vi "LV_client_23.vi"() -> ()   [LabVIEW 2022 SP3]
doc: "Demo VI, client making TCP connection with server on the local port 8089"
panel:
  out "Path to Python script":path
  out "error out":errorcluster
  in  "Stop":bool
  out "Answer":string
  in  "Ping":bool
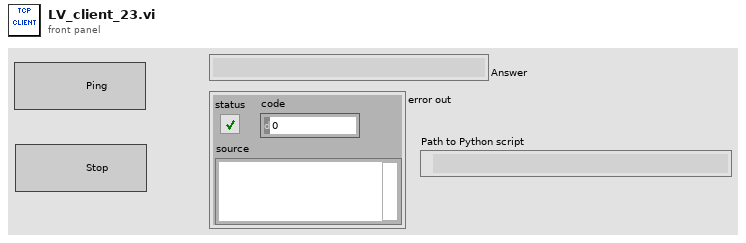
[diagram p1: front panel]
types:
  T1 = enum8{"Enabled", "Disabled", "Disabled and Grayed Out"}
  T2 = enum16{"Standard", "Buffered", "CRLF", "Immediate"}
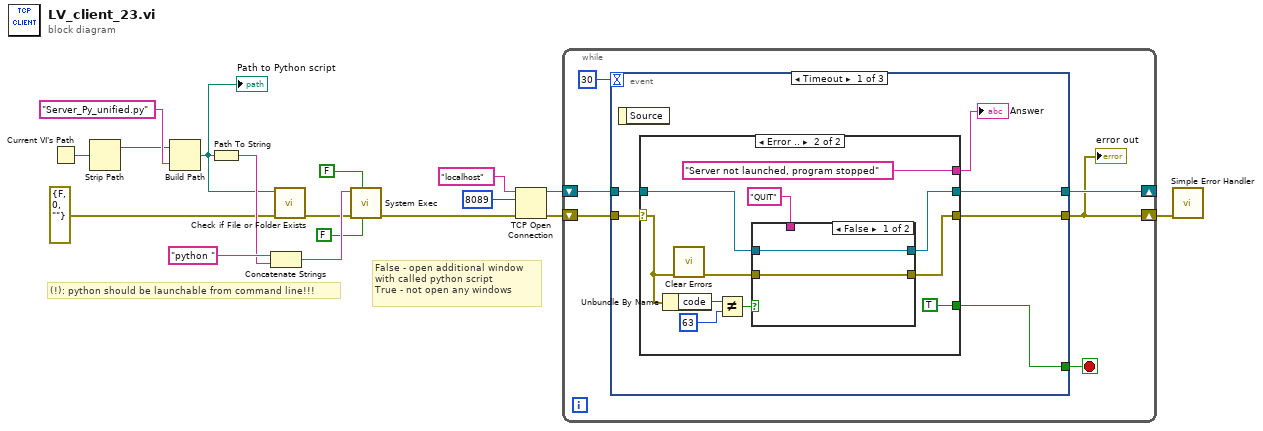
[diagram p0: block diagram]
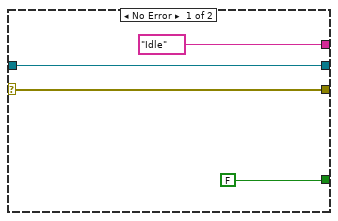
[diagram p2: hidden frame]
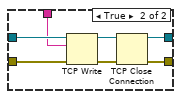
[diagram p3: hidden frame]
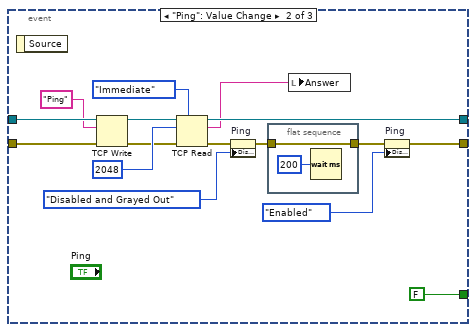
[diagram p4: hidden frame]
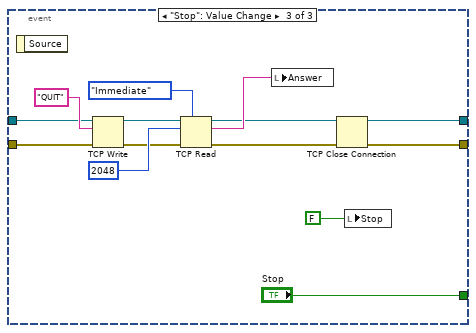
[diagram p5: hidden frame]
diagram:
  # "False - open additional window\nwith called python script\nTrue - not open any windows"
  # "(!): python should be launchable from command line!!!"
  n1 = Current VI's Path() -> (path=w12:path)
  n2 = Strip Path(path=w12) -> (stripped path=w5:path)  [unwired: 1 out]
  n3 = Build Path(base path=w5, name or relative path="Server_Py_unified.py" ("string")) -> (appended path=w3:path)
  "Path to Python script" <- w3
  n4 = Path To String(path=w3) -> (string=w6:string)
  n5 = Concatenate Strings("python " ("command line"), w6) -> (w10:string)
  n6 = call <vilib>:"Check if File or Folder Exists.vi"("error in (no error)"=errorcluster {"status"=FALSE, "code"=0, "source"=""}, "path"=w3) -> ("error out"=w2:errorcluster)  [unwired: 7 in, 2 out]
  n7 = call <vilib>:"System Exec.vi"("run minimized? (F)"=FALSE, "wait until completion? (T)"=FALSE, "error in (no error)"=w2, "command line"=w10) -> ("error out"=w9:errorcluster)  [unwired: 4 in, 3 out]
  n8 = TCP Open Connection(address="localhost", remote port or service name=u16 8089, error in (no error)=w9) -> (connection ID=w16:refnum<k5>, error out=w15:errorcluster)  [unwired: 2 in]
  n9 = while {
    shift-right: [w20] -> _
    shift-left: w16 -> [w21]
    shift-right: [w18] -> w13
    shift-left: w15 -> [w22]
    stop <- w19 stop-if-true
    n10 = event shown="[0] Timeout" {
      selector: _ -> [_ _ _]
      dyn-events: _ -> [_ _ _]
      timeout: 30 -> [_ _ _]
      tunnel: [w25 FALSE ("Stop") "Stop"] -> w19
      tunnel: w22 -> [w29 w68 w79]
      tunnel: w21 -> [w28 w69 w78]
      tunnel: [w27 w62 w73] -> w20
      tunnel: [w26 w55 w72] -> w18
      event Timeout {
        n11 = event-data() -> ()  [unwired: 1 in, 1 out]
        n12 = case shown="Error .." w29 {
          selector: w29 -> [w32 w39]
          tunnel: [w33 w41] -> w27
          tunnel: w28 -> [w33 w42]
          tunnel: [w32 w34] -> w26
          tunnel: [FALSE ("Stop") TRUE ("Stop")] -> w25
          tunnel: ["Idle" ("Answer") "Server not launched, program stopped" ("Answer")] -> w24
          frame No Error {
          }
          frame Error {
            n13 = Unbundle By Name(w39) -> ("code"=w38:i32)
            n14 = call <vilib>:"Clear Errors.vi"("error in (no error)"=w39) -> ("error out"=w44:errorcluster)  [unwired: 5 in, 1 out]
            n15 = Not Equal?(x=w38, y=63) -> (x != y?=w36:bool)
            n16 = case shown="False" w36 {
              tunnel: w44 -> [w45 w53]
              tunnel: w42 -> [w46 w52]
              tunnel: [w46 w49] -> w41
              tunnel: "QUIT" ("data in") -> [_ w48]
              tunnel: [w45 w47] -> w34
              frame False {
              }
              frame True {
                n17 = TCP Write(connection ID=w52, data in=w48, error in (no error)=w53) -> (connection ID out=w50:refnum<k5>, error out=w51:errorcluster)  [unwired: 1 in, 1 out]
                n18 = TCP Close Connection(connection ID=w50, error in (no error)=w51) -> (connection ID out=w49:refnum<k5>, error out=w47:errorcluster)  [unwired: 1 in]
              }
            }
          }
        }
        "Answer" <- w24
      }
      event "Ping": Value Change {
        n19 = event-data() -> ()  [unwired: 1 in, 1 out]
        n20 = TCP Write(connection ID=w69, data in="Ping", error in (no error)=w68) -> (connection ID out=w66:refnum<k5>, error out=w63:errorcluster)  [unwired: 1 in, 1 out]
        n21 = TCP Read(connection ID=w66, bytes to read=2048, error in (no error)=w63, 7:T2."Immediate" ("mode (standard)")) -> (connection ID out=w62:refnum<k5>, data out=w60:string, error out=w59:errorcluster)  [unwired: 1 in]
        n22 = property on="Ping" class="Bool"(error in=w59, "DisabledEnum"=T1."Disabled and Grayed Out" ("Disabled")) -> (error out=w58:errorcluster)  [unwired: 1 in, 1 out]
        n23 = flat-sequence {
          tunnel: w58 -> [w70]
          tunnel: [w70] -> w56
          frame #0 {
            n24 = Wait (ms)(milliseconds to wait=u32 200) -> ()  [unwired: 1 out]
          }
        }
        n25 = local write "Answer"(w60) -> ()
        n26 = property on="Ping" class="Bool"(error in=w56, "DisabledEnum"=T1."Enabled" ("Disabled")) -> (error out=w55:errorcluster)  [unwired: 1 in, 1 out]
      }
      event "Stop": Value Change {
        n27 = event-data() -> ()  [unwired: 1 in, 1 out]
        n28 = TCP Write(connection ID=w78, data in="QUIT", error in (no error)=w79) -> (connection ID out=w83:refnum<k5>, error out=w80:errorcluster)  [unwired: 1 in, 1 out]
        n29 = TCP Read(connection ID=w83, bytes to read=2048, error in (no error)=w80, 7:T2."Immediate" ("mode (standard)")) -> (connection ID out=w74:refnum<k5>, data out=w77:string, error out=w75:errorcluster)  [unwired: 1 in]
        n30 = local write "Answer"(w77) -> ()
        n31 = TCP Close Connection(connection ID=w74, error in (no error)=w75) -> (connection ID out=w73:refnum<k5>, error out=w72:errorcluster)  [unwired: 1 in]
        n32 = local write "Stop"(FALSE ("Stop")) -> ()
      }
    }
    "error out" <- w18
  }
  n33 = call <vilib>:"Simple Error Handler.vi"("error in (no error)"=w13) -> ()  [unwired: 4 in, 5 out]
